vi "DAQ Digital Waveform Output.vi"(8 "error in":errorcluster, 10 "Waveform":digitalwaveform(waveform)={"t0"=timestamp(0 s since 1904-01-01), "dt"=0.0, "Y"={"transitions"=[], "data"=[]}, "error"={"status"=FALSE, "code"=37421928, "source"=""}}, 11 "task/channels in":refnum<k21>) -> (0 "error out":errorcluster, 3 "task out":refnum<k21>)   [LabVIEW 2021]
uses:
  <vilib>/DAQmx/write.llb/DAQmx Write (Digital Wfm 1Chan NSamp).vi
  <vilib>/Waveform/DWDTOps.llb/DWDT Uncompress Digital.vi
  <vilib>/DAQmx/miscellaneous.llb/DAQmx Fill In Error Info.vi
panel:
  out "number of samples written per channel":u32
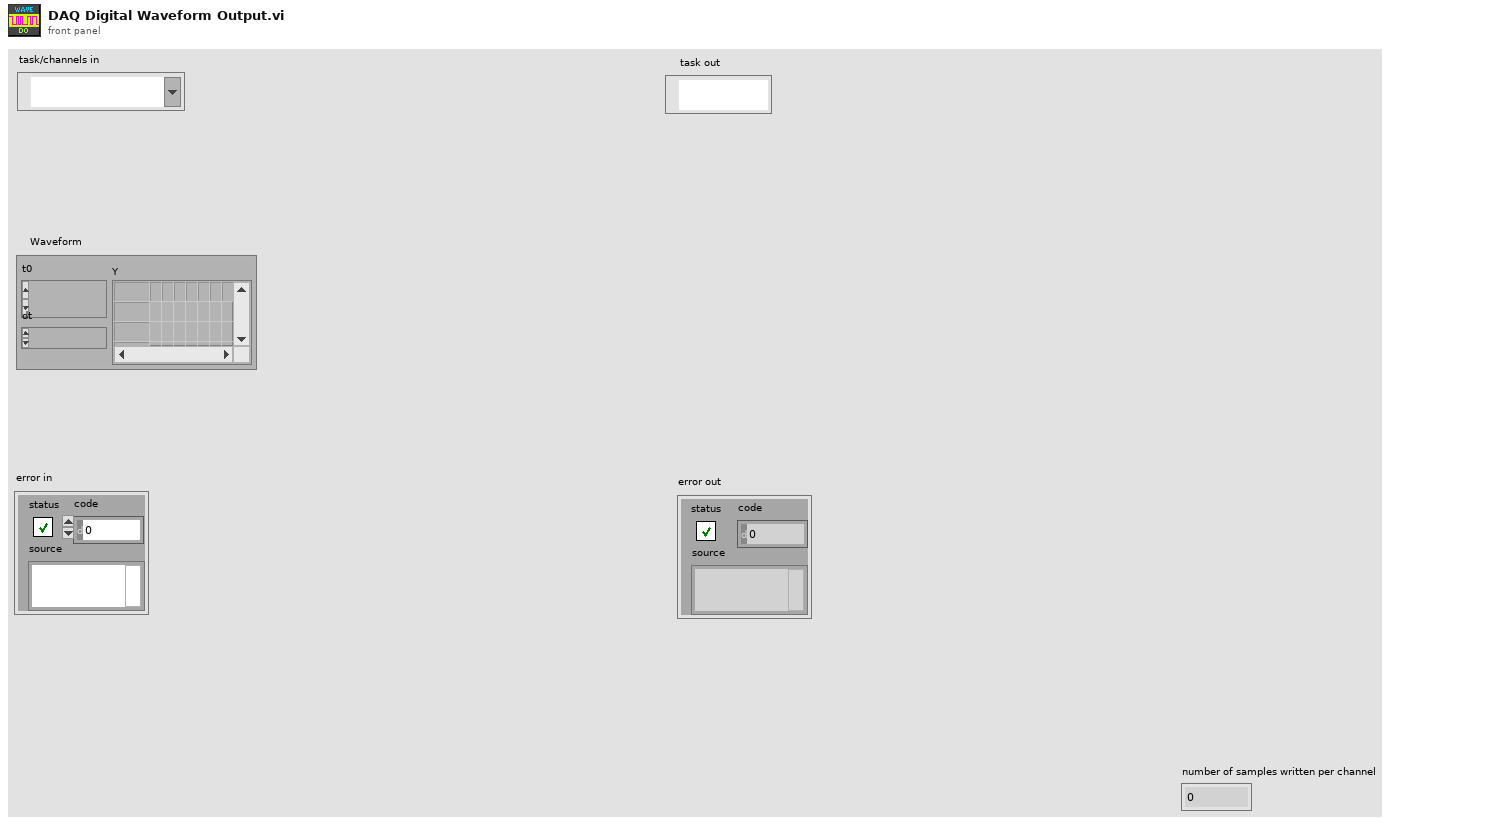
[diagram p1: front panel]
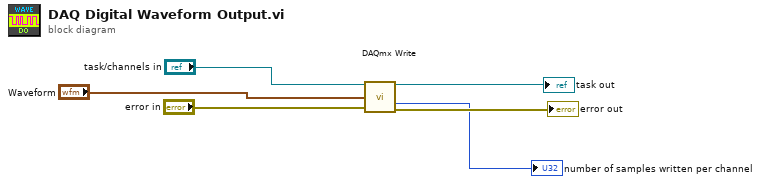
[diagram p0: block diagram]
diagram:
  n1 = call-poly <vilib>:"DAQmx Write.vi"("task/channels in"="task/channels in", "data"="Waveform", "error in"="error in") -> ("task out"=→"task out":refnum<k21>, "number of samples written per channel"=→"number of samples written per channel":u32, "error out"=→"error out":errorcluster)  [unwired: 10 in]
